vi "Dashboard Main.vi"() -> ()   [LabVIEW 2013]
uses:
  Program Files/National Instruments/LabVIEW 2013/examples/FRC/Vision/2014 Target Detection/TargetType.ctl
  <vilib>/event_ctls.llb/eventvkey.ctl
  <vilib>/Rock Robotics/WPI/Dashboard/WPI_DashboardLogging Global.vi
  <vilib>/Utility/config.llb/Write Key (String).vi
  <vilib>/Utility/config.llb/Write Key (I32).vi
  <vilib>/Utility/config.llb/NI_LVConfig.lvlib
panel:
  out "Image Message":string="Timeout in Camera Communications"
  in  "Rec Mode":enum32{"Stop", "Record", "Playback"}(radio)
  in  "Dashboard Tab":T1(tab)
  in  "Camera Settings":T2={"Frame Rate"=30, "Compression"=30, "Size"=1} {"Frame Rate" scale=1.0..30.0; "Size" items=["640x480", "320x240", "160x120"]}
  out "MotorSliders R":cluster{"MotorSlide1":dbl, "MotorSlide2":dbl} {"MotorSlide2" scale=-1.0..1.0 scale format="%#_2e"; "MotorSlide1" scale=-1.0..1.0 scale format="%#_2e"}
  out "MotorChart R":cluster{"Numeric":dbl, "Numeric":dbl}(graph)
  out "MotorSliders L":T3 {"MotorSlide4 2" scale=0.0..14.0 scale format="%#_2e"; "MotorSlide2" scale=-1.0..1.0 scale format="%#_2e"; "MotorSlide1" scale=-1.0..1.0 scale format="%#_2e"}
  out "MotorChart L":T4(graph)
  out "JS1 Z":dbl(slide) scale=-1.0..1.0 scale format="%#_2e"
  out "Joystick 1":cluster{"X":dbl, "Y":dbl}[](graph)
  out "JS Buttons 1":T5
  out "JS2 Z":dbl(slide) scale=-1.0..1.0 scale format="%#_2e"
  out "Joystick 2":cluster{"X":dbl, "Y":dbl}[](graph)
  out "JS Buttons 2":T5
  out "Mode":T6(ring)=enum."Auto Disabled"
  out "Camera IP":string
  in  "DB Camera Config":bool
  out "fps":dbl format="%#.1g"
  out "Mbps":dbl format="%#.1g"
  out "Mbps 2":bool
  out "LED 1":bool
  in  "Slider 1":dbl(slide) scale=0.0..100.0
  out "Mask":T7(plugin-control)
  out "Distances":T9(array[cluster])
  in  "Score Limit":dbl=70.0
  in  "Color Components":T10={"Hue"={110.0, 142.0}, "Sat"={138.0, 255.0}, "Val"={139.0, 198.0}} {"Val" scale=0.0..255.0; "Sat" scale=0.0..255.0; "Hue" scale=0.0..255.0 scale format="%#_3g"}
  in  "Checkbox 2":bool
  in  "Checkbox 1":bool
  in  "Test Slider":dbl(slide) scale=0.0..100.0 scale format="%#_3g"
  in  "On/Off":bool caption="Solenoid"
  in  "Test Name":u16(ring) items=["Select the test to run...", "Example Test", "-------------------------------", "List of tests is built in robot code.", "Replace with your own automated tests."]
  in  "Test Tree":string(tree)
  in  "Motor":cluster{"Value":dbl, "Enable":bool} {"Value" scale=-1.0..1.0 scale format="%#_3g"}
  out "Progress":T11 {"Test Progress" scale=0.0..100.0}
  in  "Rev/Fwd":cluster{"Forward":bool, "Reverse":bool}
  in  "Test Ring":u16(ring) items=["Auto", "Fixed indoor", "Fixed outdoor 1", "Fixed outdoor 2", "Fixed fluorescent 1", "Fixed fluorescent 2", "Hold current"]
  in  "Listbox":i32(listbox)
  out "Tree":string(tree)
  out "Camera Image":T7(plugin-control)
  in  "Enable":bool
  # "Left"
  # "Front"
  # "Right"
  # "Battery"
  # "Customize by placing controls and indicators here and name to\nmatch Dashboard Variables on robot."
  # "This tab is a great place for autonomous settings and validation.\nCustomize by placing controls and indicators here and name to\nmatch Dashboard Variables on robot."
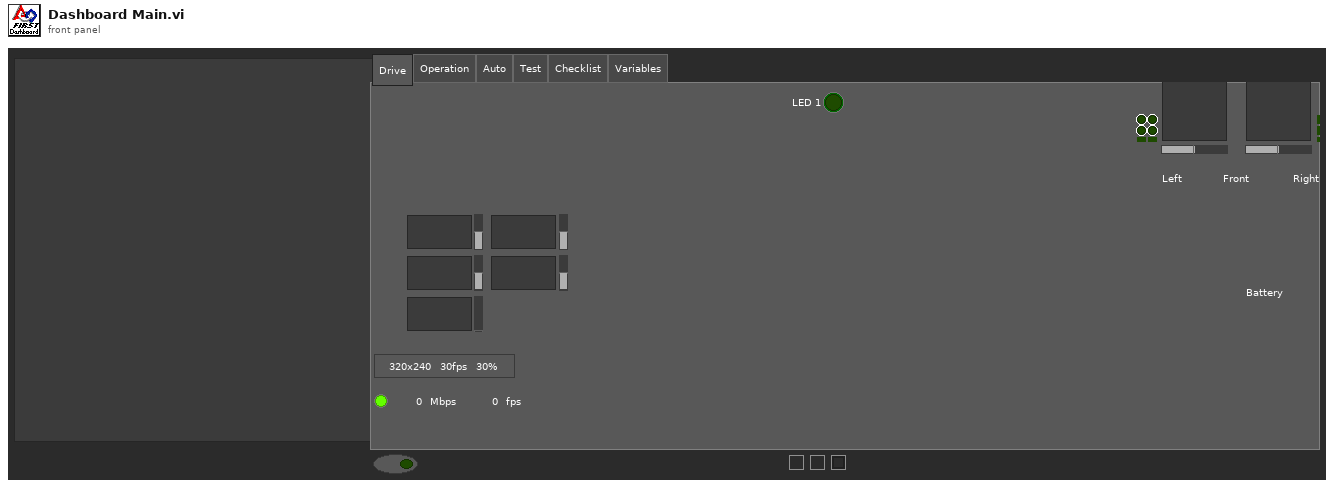
[diagram p1: front panel]
types:
  T1 = enum32{"Drive", "Operation", "Auto", "Test", "Checklist", "Variables"}
  T2 = cluster{"Frame Rate":i32, "Compression":i32, "Size":u16}
  T3 = cluster{"MotorSlide1":dbl, "MotorSlide2":dbl, "MotorSlide4 2":dbl}
  T4 = cluster{"Numeric":dbl, "Numeric":dbl, "Battery":sgl}
  T5 = cluster{bool, bool, bool, bool, bool, bool, bool, bool, bool, bool, bool, bool}
  T6 = enum8{"Tele-Op Disabled", "Tele-Op Enabled", "Auto Disabled", "Auto Enabled", "Test Disabled", "Test Enabled", ""}
  T7 = typedef "IMAQ Image.ctl" = refnum<image>
  T8 = typedef "TargetType.ctl" = enum16{"Not Hot", "Hot"}
  T9 = cluster{"Distance (ft)":dbl, "Target Center (-1 to 1)":cluster{"X":dbl, "Y":dbl}, "Left":bool, "State":T8}[]
  T10 = cluster{"Hue":cluster{dbl, dbl}, "Sat":cluster{dbl, dbl}, "Val":cluster{dbl, dbl}}
  T11 = cluster{"Test Progress":u8, "Test Progress Text":string}
  T12 = typedef "Image Type" = u32
  T13 = cluster{"Horizontal":bool, "Aspect Score":dbl, "Rect Score":dbl, cluster{"Left":dbl, "Top":dbl, "Right":dbl, "Bottom":dbl}, "Equiv H":dbl, "Equiv V":dbl}[]
  T14 = cluster{"Scores":cluster{"Total":dbl, "Left":dbl, "Right":dbl, "Ratio":dbl, "Vertical":dbl, "index":i32, "State":T8}, "Verticals":cluster{"Horizontal?":bool, "Aspect Score":dbl, "Rect Score":dbl, cluster{"Left":dbl, "Top":dbl, "Right":dbl, "Bottom":dbl}, "Equiv H":dbl, "Equiv V":dbl}, "Horizontals":cluster{"Horizontal?":bool, "Aspect Score":dbl, "Rect Score":dbl, cluster{"Left":dbl, "Top":dbl, "Right":dbl, "Bottom":dbl}, "Equiv H":dbl, "Equiv V":dbl}, "Validated":bool}[]
  T15 = cluster{cluster{dbl, dbl}, cluster{dbl, dbl}, cluster{dbl, dbl}}
  T16 = cluster{"Digital Inputs":bool[], "Digital Outputs":bool[]}
  T17 = cluster{"Competition mode":bool, "Robot Link":bool, "Autonomous":bool, "Enabled":bool, "E-Stop":bool, "Simulated":bool, "TestMode":bool, "Docked Window":bool}
  T18 = cluster{"Boolean Array[0]":bool, "Boolean Array[1]":bool, "Boolean Array[2]":bool, "Boolean Array[3]":bool, "Boolean Array[4]":bool, "Boolean Array[5]":bool, "Boolean Array[6]":bool, "Boolean Array[7]":bool, "Boolean Array[8]":bool, "Boolean Array[9]":bool, "Boolean Array[10]":bool, "Boolean Array[11]":bool}
  T19 = typedef "NI_LVConfig.lvlib/Config Data RefNum.ctl" = refnum<k1>
  T20 = typedef "eventvkey.ctl" = enum16{"ASCII", "Enter", "Return", "Shift", "Ctrl", "Alt", "Cmd", "Opt", "Caps", "NumLock", "Clear", "Break", "Up", "Down", "Left", "Right", "Insert", "Delete", "Home", "End", "PageUp", "PageDown", "Escape", "Help", "Pause", "ScrollLock", "F1", "F2", "F3", "F4", "F5", "F6", "F7", "F8", "F9", "F10", "F11", "F12", "F13", "F14", "F15", "F16", "F17", "F18", "F19", "F20", "F21", "F22", "F23", "F24", "Play", "VolumeUp", "VolumeDown", "Mute", "Two Byte Char"}
  T21 = cluster{"Image Size":bool, "Image Type":bool, "Pixel Value":bool, "ROI Information":bool, "Zoom Factor":bool}
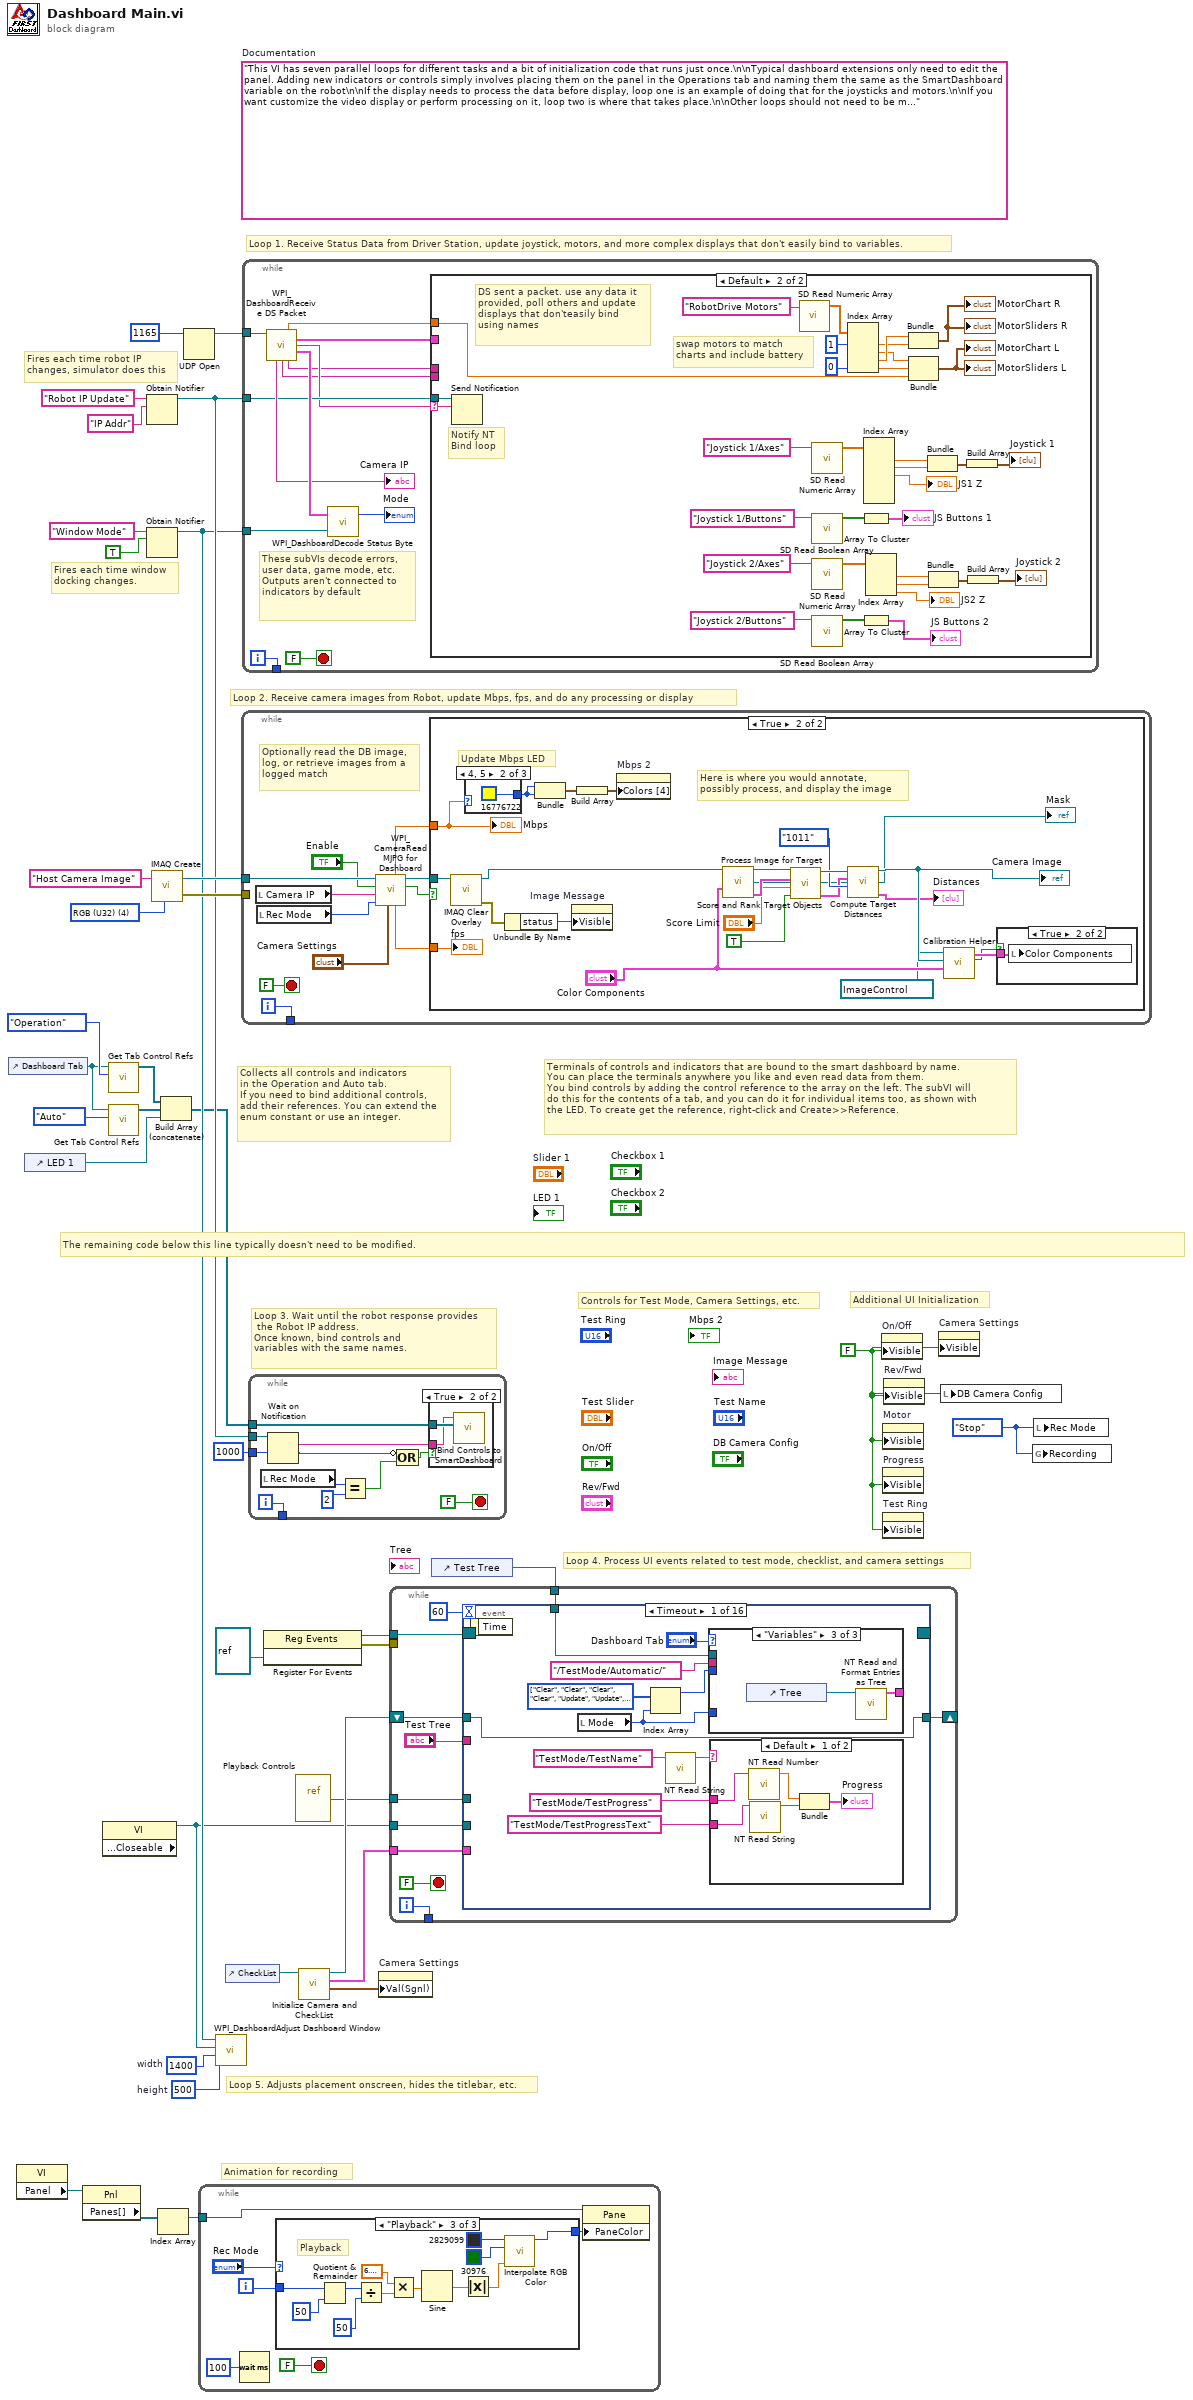
[diagram p0: block diagram]
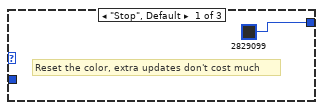
[diagram p2: hidden frame]
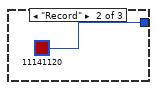
[diagram p3: hidden frame]
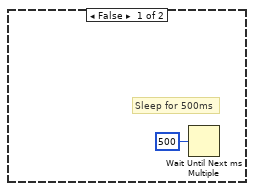
[diagram p5: hidden frame]
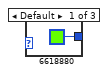
[diagram p7: hidden frame]
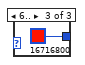
[diagram p8: hidden frame]
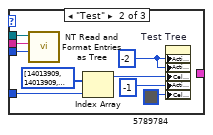
[diagram p10: hidden frame]
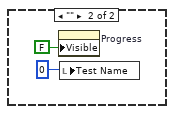
[diagram p11: hidden frame]
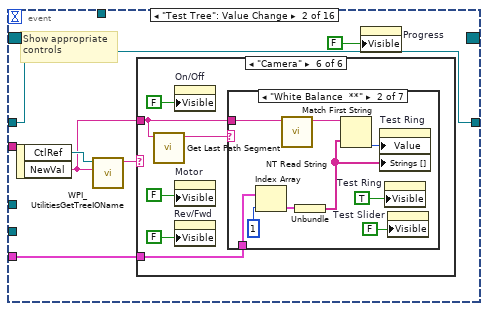
[diagram p12: hidden frame]
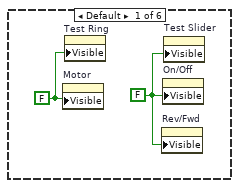
[diagram p13: hidden frame]
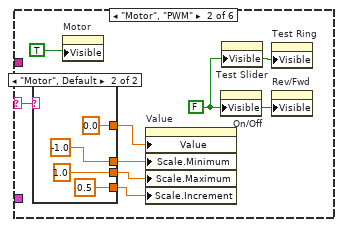
[diagram p14: hidden frame]
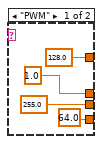
[diagram p15: hidden frame]
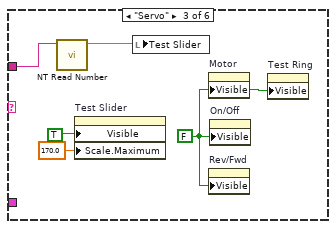
[diagram p16: hidden frame]
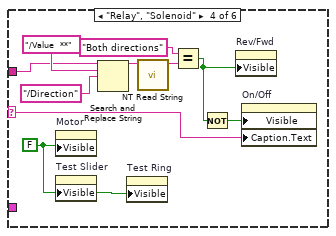
[diagram p17: hidden frame]
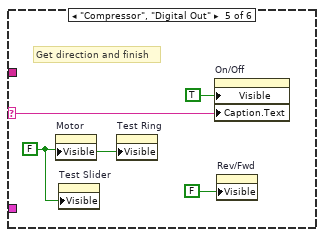
[diagram p18: hidden frame]
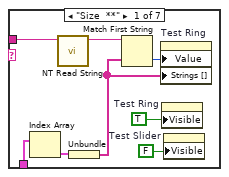
[diagram p19: hidden frame]
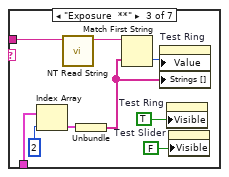
[diagram p20: hidden frame]
diagram:
  w8 = enum32{"Stop", "Record", "Playback"}."Stop" ("Rec Mode")
  w11 = 500  # height
  w12 = 1400  # width
  w25 = FALSE ("Visible")
  (unwired) "This VI has seven parallel loops for different tasks and a bit of initialization code that runs just once.\n\nTypical dashboard extensions only need to edit the panel. Adding new indicators or controls simply involves placing them on the panel in the Operations tab and naming them the same as the SmartDashboard variable on the robot\n\nIf the display needs to process the data before display, loop one is an example of doing that for the joysticks and motors.\n\nIf you want customize the video display or perform processing on it, loop two is where that takes place.\n\nOther loops should not need to be modified. They are pretty standard, and document the task they perform."  # Documentation
  w35 = T12 4 items=["Grayscale (U8)", "Grayscale (I16)", "Grayscale (SGL)", "Complex (CSG)", "RGB (U32)", "HSL (U32)", "RGB (U64)"] ("Image Type")
  # "Controls for Test Mode, Camera Settings, etc."
  # "Additional UI Initialization"
  # "Animation for recording"
  # "Fires each time robot IP\nchanges, simulator does this"
  # "Fires each time window\ndocking changes."
  # "Collects all controls and indicators\nin the Operation and Auto tab.\nIf you need to bind additional controls,\nadd their references. You can extend the\nenum constant or use an integer."
  # "The remaining code below this line typically doesn't need to be modified."
  # "Loop 4. Process UI events related to test mode, checklist, and camera settings"
  # "Terminals of controls and indicators that are bound to the smart dashboard by name.\nYou can place the terminals anywhere you like and even read data from them.\nYou bind controls by adding the control reference to the array on the left. The subVI will\ndo this for the contents of a tab, and you can do it for individual items too, as shown with\nthe LED. To create get the reference, right-click and Create>>Reference."
  # "Loop 3. Wait until the robot response provides\n the Robot IP address.\nOnce known, bind controls and\nvariables with the same names."
  # "Loop 5. Adjusts placement onscreen, hides the titlebar, etc."
  # "Loop 1. Receive Status Data from Driver Station, update joystick, motors, and more complex displays that don't easily bind to variables."
  # "Loop 2. Receive camera images from Robot, update Mbps, fps, and do any processing or display"
  n1 = control-ref of="Dashboard Tab"() -> (w6:refnum<vi>)
  n2 = property class="VI"() -> ("Panel"=w19:refnum<vi>)  [unwired: 2 in, 2 out]
  n3 = control-ref of="LED 1"() -> (w1:refnum<vi>)
  n4 = property class="Pnl"(reference=w19) -> ("Panes[]"=w20:refnum<vi>[])  [unwired: 1 in, 2 out]
  n5 = property class="VI" props=["Front Panel.Closeable"]() -> (reference out=w7:refnum<vi>)  [unwired: 2 in, 2 out]
  n6 = call <vilib>:"Get Tab Control Refs.vi"("Page Index"=T1."Operation" ("Dashboard Tab"), "TabControl in"=w6) -> ("ControlsOnPage"=w4:refnum<vi>[])  [unwired: 9 in]
  n7 = call <vilib>:"Get Tab Control Refs.vi"("Page Index"=T1."Auto" ("Dashboard Tab"), "TabControl in"=w6) -> ("ControlsOnPage"=w5:refnum<vi>[])  [unwired: 9 in]
  n8 = Obtain Notifier(name (unnamed)="Robot IP Update", notification data type="IP Addr" ("name (unnamed)")) -> (notifier out=w29:refnum<notifier>)  [unwired: 2 in, 2 out]
  n9 = Obtain Notifier(name (unnamed)="Window Mode", notification data type=TRUE) -> (notifier out=w10:refnum<notifier>)  [unwired: 2 in, 2 out]
  n10 = call "IMAQ Create"("Image Name"="Host Camera Image", "Image Type"=w35) -> ("New Image"=w33:T7, "error out"=w32:errorcluster)  [unwired: 2 in, 1 out]
  n11 = Index Array(array=w20) -> (element=w18:refnum<vi>)  [unwired: 1 in]
  n12 = Build Array (concatenate)(w4, w5, w1) -> (w3:refnum<vi>[])
  n13 = UDP Open(11:u16 1165 ("port")) -> (port=w36:refnum<k16>)  [unwired: 2 in, 4 out]
  n14 = while {
    tunnel: w18 -> [w39]
    i -> [w42]
    stop <- FALSE stop-if-true
    n15 = Wait (ms)(milliseconds to wait=u32 100) -> ()  [unwired: 1 out]
    n16 = case shown="\"Playback\"" "Rec Mode" {
      tunnel: w42 -> [_ _ w57]
      tunnel: [u32 2829099 ("Base Color") u32 11141120 ("Target Color") w46] -> w38
      frame "Stop", Default {
        # "Reset the color, extra updates don't cost much"
      }
      frame "Record" {
      }
      frame "Playback" {
        # "Playback"
        n17 = Quotient & Remainder(x=w57, y=u32 50 ("milliseconds to wait")) -> (x-y*floor(x/y)=w53:u32)  [unwired: 1 out]
        n18 = Divide(x=w53, y=u32 50 ("milliseconds to wait")) -> (x/y=w50:dbl)
        n19 = Multiply(x=6.283185307179586, y=w50) -> (x*y=w55:dbl)
        n20 = Sine(x=w55) -> (sin(x)=w54:dbl)
        n21 = Absolute Value(x=w54) -> (abs(x)=w47:dbl)
        n22 = call "Interpolate RGB Color.vi"("Proportion"=w47, "Target Color"=u32 30976, "Base Color"=u32 2829099) -> ("Result Color"=w46:u32)  [unwired: 8 in]
      }
    }
    n23 = property class="Pane"(reference=w39, "PaneColor"=w38) -> ()  [unwired: 1 in, 2 out]
  }
  n24 = call <vilib>:"WPI_DashboardAdjust Dashboard Window.vi"("height"=w11, "width"=w12, "reference in"=w7, "Notifier in"=w10) -> ()  [unwired: 8 in]
  n25 = control-ref of="CheckList"() -> (w9:refnum<vi>)
  n26 = while {
    tunnel: w33 -> [w66]
    tunnel: w32 -> [_]
    tunnel: [w67] -> _
    i -> [w67]
    stop <- FALSE stop-if-true
    # "Optionally read the DB image,\nlog, or retrieve images from a\nlogged match"
    n27 = local read "Camera IP"() -> (w59:string)
    n28 = local read "Rec Mode"() -> (w58:enum32{"Stop", "Record", "Playback"})
    n29 = call <vilib>:"WPI_CameraRead MJPG for Dashboard.vi"("Camera Settings"="Camera Settings", "Rec Mode"=w58, "Camera IP"=w59, "Enable"="Enable", "Refnum in"=w66) -> ("Active"=w63:bool, "Refnum out"=w65:T7, "FPS"=w62:dbl, "Bandwidth (Mbps)"=w61:dbl)  [unwired: 3 in]
    n30 = case shown="True" w63 {
      tunnel: w65 -> [_ w87]
      tunnel: w61 -> [_ w86]
      tunnel: w62 -> [_ w85]
      frame False {
        # "Sleep for 500ms"
        n31 = Wait Until Next ms Multiple(millisecond multiple=u32 500) -> ()  [unwired: 1 out]
      }
      frame True {
        # "Here is where you would annotate,\npossibly process, and display the image"
        # "Update Mbps LED"
        n32 = call "IMAQ Clear Overlay"("Image"=w87) -> ("error out"=w91:errorcluster, "Image Out"=w84:T7)  [unwired: 2 in, 7 out]
        n33 = case shown="4, 5" w86 {
          tunnel: [u32 6618880 ("Color Box") u32 16776722 ("Color Box") u32 16716800 ("Color Box")] -> w88
          frame Default {
          }
          frame 4, 5 {
          }
          frame 6.. {
          }
        }
        n34 = Unbundle By Name(w91) -> ("status"=w92:bool)
        n35 = Bundle("Color Box"=w88, "Color Box"=w88) -> (w90:cluster{"Color Box":u32, "Color Box":u32})  [unwired: 1 out]
        n36 = property on="Image Message" class="Str"("Visible"=w92) -> ()  [unwired: 2 in, 2 out]
        n37 = Build Array(w90) -> (w89:cluster{"Color Box":u32, "Color Box":u32}[])
        n38 = property on="Mbps 2" class="Bool (strict)"("Colors [4]"=w89) -> ()  [unwired: 2 in, 2 out]
        n39 = call "Process Image for Target.vi"("Src Image"=w84, "Color Components"="Color Components") -> ("Src Image Out"=w83:T7, "Threshold"=→"Mask":T7, "Particles"=w78:T13)  [unwired: 11 in]
        n40 = call "Score and Rank Target Objects.vi"("Annotate"=TRUE, "Score Limit"="Score Limit", "Particles"=w78, "Image in"=w83) -> ("Target Info"=w73:T14, "Annotated Image"=w82:T7)  [unwired: 6 in]
        n41 = call "Compute Target Distances.vi"("Camera Type"=enum16{"206", "1011", "1013"}."1011", "Target Info"=w73, "Image in"=w82) -> ("Distances"=→"Distances":T9, "Image out"=w81:T7)  [unwired: 6 in, 1 out]
        "Camera Image" <- w81
        n42 = call "Calibration Helper.vi"("Color Components"="Color Components", "Image"=w81, "Image Ctl Refnum"=refnum<vi> refnum) -> ("Changed"=w71:bool, "output color"=w79:T15)  [unwired: 7 in]
        n43 = case shown="True" w71 {
          tunnel: w79 -> [_ w93]
          frame False {
          }
          frame True {
            n44 = local write "Color Components"(w93) -> ()
          }
        }
        "Mbps" <- w86
        "fps" <- w85
      }
    }
  }
  n45 = while {
    tunnel: w36 -> [w107]
    tunnel: w29 -> [w102]
    tunnel: w10 -> [w106]
    tunnel: [w103] -> _
    i -> [w103]
    stop <- FALSE stop-if-true
    # "These subVIs decode errors, user data, game mode, etc.\nOutputs aren't connected to indicators by default"
    n46 = call <vilib>:"WPI_DashboardReceive DS Packet.vi"("Recv Socket"=w107) -> ("Battery"=w97:sgl, "Driver Station"=w98:T16, "Robot IP Address"=w101:string, "Status"=w108:T17, "Camera IP Address"=→"Camera IP":string, "Low Priority User Data"=w100:string, "High Priority User Data"=w99:string)  [unwired: 1 in, 7 out]
    n47 = call <vilib>:"WPI_DashboardDecode Status Byte.vi"("Window Mode Notifier"=w106, "Status"=w108) -> ("Mode"=→"Mode":T6)  [unwired: 1 out]
    n48 = case shown="Default" w101 {
      selector: w101 -> [_ w120]
      tunnel: w102 -> [_ w121]
      tunnel: w100 -> [_ _]
      tunnel: w99 -> [_ _]
      tunnel: w98 -> [_ _]
      tunnel: w97 -> [_ w119]
      frame "0.0.0.0" {
        # "DS not sending packets, or no robot exists yet.\nDon't poll the variables"
      }
      frame Default {
        # "Notify NT\nBind loop"
        # "DS sent a packet. use any data it\nprovided, poll others and update\ndisplays that don'teasily bind\nusing names"
        # "swap motors to match\ncharts and include battery"
        n49 = Send Notification(notification=w120, notifier=w121) -> ()  [unwired: 1 in, 2 out]
        n50 = call <vilib>:"SD Read Numeric Array.vi"("Name"="RobotDrive Motors") -> ("Numeric Array"=w118:dbl[])  [unwired: 8 in, 2 out]
        n51 = call <vilib>:"SD Read Numeric Array.vi"("Name"="Joystick 1/Axes") -> ("Numeric Array"=w137:dbl[])  [unwired: 8 in, 2 out]
        n52 = call <vilib>:"SD Read Boolean Array.vi"("Name"="Joystick 1/Buttons") -> ("Boolean Array"=w139:bool[])  [unwired: 8 in, 2 out]
        n53 = call <vilib>:"SD Read Numeric Array.vi"("Name"="Joystick 2/Axes") -> ("Numeric Array"=w131:dbl[])  [unwired: 8 in, 2 out]
        n54 = call <vilib>:"SD Read Boolean Array.vi"("Name"="Joystick 2/Buttons") -> ("Boolean Array"=w130:bool[])  [unwired: 8 in, 2 out]
        n55 = Index Array(array=w118, index #1=1, index #4=0) -> (element #1=w114:dbl, element #2=w113:dbl, element #3=w115:dbl, element #4=w110:dbl)  [unwired: 2 in]
        n56 = Array To Cluster(array=w139) -> (cluster=→"JS Buttons 1":T18)
        n57 = Array To Cluster(array=w130) -> (cluster=→"JS Buttons 2":T18)
        n58 = Index Array(array=w137) -> (element #1=w134:dbl, element #2=w135:dbl, element #3=→"JS1 Z":dbl)  [unwired: 6 in, 3 out]
        n59 = Index Array(array=w131) -> (element #1=w126:dbl, element #2=w125:dbl, element #3=→"JS2 Z":dbl)  [unwired: 3 in]
        n60 = Bundle("Numeric"=w115, "Numeric"=w114) -> (→"MotorChart R" →"MotorSliders R":cluster{"Numeric":dbl, "Numeric":dbl})  [unwired: 1 in]
        n61 = Bundle("Numeric"=w113, "Numeric"=w110, "Battery"=w119) -> (→"MotorChart L" →"MotorSliders L":T4)  [unwired: 1 in]
        n62 = Bundle("Numeric"=w134, "Numeric"=w135) -> (w133:cluster{"Numeric":dbl, "Numeric":dbl})  [unwired: 1 in]
        n63 = Bundle("Numeric"=w126, "Numeric"=w125) -> (w127:cluster{"Numeric":dbl, "Numeric":dbl})  [unwired: 1 in]
        n64 = Build Array(w133) -> (→"Joystick 1":cluster{"Numeric":dbl, "Numeric":dbl}[])
        n65 = Build Array(w127) -> (→"Joystick 2":cluster{"Numeric":dbl, "Numeric":dbl}[])
      }
    }
  }
  n66 = while {
    tunnel: w3 -> [w153]
    tunnel: w29 -> [w151]
    tunnel: [w149] -> _
    tunnel: u32 1000 ("milliseconds to wait") -> [w148]
    i -> [w149]
    stop <- FALSE stop-if-true
    n67 = local read "Rec Mode"() -> (w144:enum32{"Stop", "Record", "Playback"})
    n68 = Wait on Notification(notifier=w151, timeout in ms (-1)=w148) -> (notification=w150:string, timed out?=w146:bool)  [unwired: 2 in, 2 out]
    n69 = Equal?(x=w144, y=u16 2 ("Rec Mode")) -> (x = y?=w145:bool)
    n70 = Compound Arithmetic op=OR(invert w146, w145) -> (w147:bool)
    n71 = case shown="True" w147 {
      tunnel: w153 -> [_ w155]
      tunnel: w150 -> [_ w154]
      frame False {
      }
      frame True {
        n72 = call <vilib>:"Bind Controls to SmartDashboard.vi"("Bound Control Refs"=w155, "Server IP Address"=w154) -> ()  [unwired: 10 in]
      }
    }
  }
  n73 = register-events(refnum<vi> refnum) -> (reference out=w16:refnum<event-registration>, error out=w15:errorcluster)  [unwired: 2 in]
  n74 = vi-ref "Playback Controls.vi"() -> (w17:refnum<vi>)
  n75 = call "Initialize Camera and CheckList.vi"("ListBox in"=w9) -> ("Cluster"=w23:cluster{"value":i32, "value":i32, "index":i32}, "Array"=w24:cluster{string[]}[], "File Refnum"=w22:T19)  [unwired: 8 in]
  n76 = property on="Camera Settings" class="Clust (strict)"("Val(Sgnl)"=w23) -> ()  [unwired: 2 in, 2 out]
  n77 = control-ref of="Test Tree"() -> (w21:refnum<vi>)
  n78 = while {
    tunnel: w24 -> [w163]
    shift-right: [w162] -> _
    shift-left: w22 -> [w161]
    tunnel: [w160] -> _
    tunnel: w21 -> [w159]
    tunnel: w17 -> [w158]
    tunnel: w16 -> [w157]
    tunnel: w15 -> [_]
    tunnel: w7 -> [w156]
    i -> [w160]
    stop <- FALSE stop-if-true
    n79 = event shown="[0] Timeout" {
      selector: w157 -> [_ _ _ _ _ _ _ _ _ _ _ _ _ _ _ _]
      dyn-events: [_ _ _ _ _ _ _ _ _ _ _ _ _ w401 _ _] -> _
      timeout: u32 60 ("milliseconds to wait") -> [_ _ _ _ _ _ _ _ _ _ _ _ _ _ _ _]
      tunnel: w159 -> [w173 _ _ _ _ _ _ _ _ _ _ _ _ _ _ _]
      tunnel: "Test Tree" -> [_ _ _ _ _ _ _ _ w370 w378 w380 w384 w392 _ _ _]
      tunnel: w163 -> [_ w197 _ _ _ _ w334 w364 _ _ _ _ _ _ _ _]
      tunnel: [w167 w196 w295 w300 w308 w320 w333 w357 w369 w376 w379 w383 w391 w403 w417 w418] -> w162
      tunnel: w161 -> [w167 w196 w295 w300 w308 w320 w332 w357 w369 w376 w379 w383 w391 w403 w417 w418]
      tunnel: w158 -> [_ _ _ _ _ _ _ _ _ _ _ _ _ w404 _ w421]
      tunnel: w156 -> [_ _ _ _ _ _ _ _ _ _ _ _ _ w399 _ _]
      event Timeout {
        w172 = enum16{"Update", "Clear"}[] [enum."Clear", enum."Clear", enum."Clear", enum."Clear", enum."Update", enum."Update", enum."Clear"] items=["Update", "Clear"]
        n80 = event-data() -> ()  [unwired: 1 in, 1 out]
        n81 = local read "Mode"() -> (w170:T6)
        n82 = Index Array(array=w172, index=w170) -> (element=w171:enum16{"Update", "Clear"})
        n83 = call <vilib>:"NT Read String.vi"("Name"="TestMode/TestName") -> ("String"=w176:string)  [unwired: 9 in, 1 out]
        n84 = case shown="\"Variables\"" "Dashboard Tab" {
          tunnel: w173 -> [_ w186 _]
          tunnel: "/TestMode/Automatic/" ("Name Pattern") -> [_ w185 _]
          tunnel: w171 -> [_ w184 _]
          tunnel: w170 -> [_ w182 _]
          tunnel: [_ _ w188] -> _
          frame "Operation", Default {
          }
          frame "Test" {
            w181 = -2 ("Active Item:Row Number")
            n85 = call <vilib>:"NT Read and Format Entries as Tree.vi"("Operation"=w184, "Name Pattern"=w185, "Tree Refnum"=w186) -> ()  [unwired: 7 in, 2 out]
            n86 = Index Array(array=u32[] [14013909, 14013909, 14013909, 14013909, 14013909, 16777215, 14013909], index=w182) -> (element=w180:u32)
            n87 = property on="Test Tree" class="Tree (strict)"("Active Item Row Number"=w181, "ActiveColNum"=w181, "CellBG"=w180, "Active Item Row Number"=-1 ("Active Item:Row Number"), "CellBG"=u32 5789784 ("Color Box")) -> ()  [unwired: 2 in, 2 out]
          }
          frame "Variables" {
            n88 = control-ref of="Tree"() -> (w187:refnum<vi>)
            n89 = call <vilib>:"NT Read and Format Entries as Tree.vi"("Tree Refnum"=w187) -> ("Formatted Strings"=w188:cluster{"Name":string, "Value":string}[])  [unwired: 9 in, 1 out]
          }
        }
        n90 = case shown="Default" w176 {
          tunnel: "TestMode/TestProgress" ("Name") -> [w190 _]
          tunnel: "TestMode/TestProgressText" ("Name") -> [w189 _]
          frame Default {
            n91 = call <vilib>:"NT Read Number.vi"("Name"=w190) -> ("Numeric"=w191:dbl)  [unwired: 9 in, 1 out]
            n92 = call <vilib>:"NT Read String.vi"("Name"=w189) -> ("String"=w192:string)  [unwired: 9 in, 1 out]
            n93 = Bundle("Numeric"=w191, "String"=w192) -> (→"Progress":cluster{"Numeric":dbl, "String":string})  [unwired: 1 in]
          }
          frame "" {
            n94 = property on="Progress" class="Clust (strict)"("Visible"=FALSE) -> ()  [unwired: 2 in, 2 out]
            n95 = local write "Test Name"(u16 0) -> ()
          }
        }
      }
      event "Test Tree": Value Change {
        # "Show appropriate\ncontrols"
        n96 = event-data() -> ("CtlRef"=w200:refnum<vi>, "NewVal"=w198:string)  [unwired: 1 in]
        n97 = call <vilib>:"WPI_UtilitiesGetTreeIOName.vi"("NewVal"=w198, "TreeControl in"=w200) -> ("I/O Name"=w201:string)  [unwired: 9 in]
        n98 = case shown="\"Camera\"" w201 {
          selector: w201 -> [_ w208 _ w226 w235 _]
          tunnel: w198 -> [_ _ w223 w225 _ w242]
          tunnel: w197 -> [_ _ _ _ _ w241]
          frame Default {
            w203 = FALSE ("Visible")
            w202 = FALSE ("Visible")
            n99 = property on="Motor" class="Clust (strict)"("Visible"=w202) -> ()  [unwired: 2 in, 2 out]
            n100 = property on="Test Ring" class="Ring (strict)"("Visible"=w202) -> ()  [unwired: 2 in, 2 out]
            n101 = property on="Rev/Fwd" class="Clust (strict)"("Visible"=w203) -> ()  [unwired: 2 in, 2 out]
            n102 = property on="On/Off" class="Bool (strict)"("Visible"=w203) -> ()  [unwired: 2 in, 2 out]
            n103 = property on="Test Slider" class="Slide (strict)"("Visible"=w203) -> ()  [unwired: 2 in, 2 out]
          }
          frame "Motor", "PWM" {
            w209 = FALSE ("Visible")
            n104 = case shown="\"Motor\", Default" w208 {
              tunnel: [1.0 ("Value") -1.0 ("Value")] -> w207
              tunnel: [255.0 ("Value") 1.0 ("Value")] -> w206
              tunnel: [128.0 ("Value") 0.0 ("Value")] -> w205
              tunnel: [64.0 ("Value") 0.5 ("Value")] -> w204
              frame "PWM" {
              }
              frame "Motor", Default {
              }
            }
            n105 = property on="Motor" class="Clust (strict)"("Visible"=TRUE) -> ()  [unwired: 2 in, 2 out]
            n106 = property on="Value" class="Slide (strict)"("Value"=w205, "Scale.Minimum"=w207, "Scale.Maximum"=w206, "Scale.Increment"=w204) -> ()  [unwired: 2 in, 2 out]
            n107 = property on="On/Off" class="Bool (strict)"("Visible"=w209) -> ()  [unwired: 2 in, 2 out]
            n108 = property on="Test Slider" class="Slide (strict)"("Visible"=w209) -> ()  [unwired: 2 in, 2 out]
            n109 = property on="Test Ring" class="Ring (strict)"("Visible"=w209) -> ()  [unwired: 2 in, 2 out]
            n110 = property on="Rev/Fwd" class="Clust (strict)"("Visible"=w209) -> ()  [unwired: 2 in, 2 out]
          }
          frame "Servo" {
            w221 = FALSE ("Visible")
            n111 = call <vilib>:"NT Read Number.vi"("Name"=w223) -> ("Numeric"=w222:dbl)  [unwired: 9 in, 1 out]
            n112 = property on="Test Slider" class="Slide (strict)"("Visible"=TRUE, "Scale.Maximum"=170.0 ("Scale.Range:Maximum")) -> ()  [unwired: 2 in, 2 out]
            n113 = local write "Test Slider"(w222) -> ()
            n114 = property on="Motor" class="Clust (strict)"("Visible"=w221) -> ()  [unwired: 2 in, 2 out]
            n115 = property on="Rev/Fwd" class="Clust (strict)"("Visible"=w221) -> ()  [unwired: 2 in, 2 out]
            n116 = property on="On/Off" class="Bool (strict)"("Visible"=w221) -> ()  [unwired: 2 in, 2 out]
            n117 = property on="Test Ring" class="Ring (strict)"("Visible"=w221) -> ()  [unwired: 2 in, 2 out]
          }
          frame "Relay", "Solenoid" {
            w224 = FALSE ("Visible")
            n118 = property on="Motor" class="Clust (strict)"("Visible"=w224) -> ()  [unwired: 2 in, 2 out]
            n119 = property on="Test Slider" class="Slide (strict)"("Visible"=w224) -> ()  [unwired: 2 in, 2 out]
            n120 = Search and Replace String(input string=w225, search string="/Value  **", replace string="/Direction") -> (result string=w231:string)  [unwired: 5 in, 3 out]
            n121 = property on="Test Ring" class="Ring (strict)"("Visible"=w224) -> ()  [unwired: 2 in, 2 out]
            n122 = call <vilib>:"NT Read String.vi"("Name"=w231) -> ("String"=w229:string)  [unwired: 9 in, 1 out]
            n123 = Equal?(x="Both directions", y=w229) -> (x = y?=w227:bool)
            n124 = Not(x=w227) -> (.not. x?=w228:bool)
            n125 = property on="Rev/Fwd" class="Clust (strict)"("Visible"=w227) -> ()  [unwired: 2 in, 2 out]
            n126 = property on="On/Off" class="Bool (strict)"("Visible"=w228, "Caption.Text"=w226) -> ()  [unwired: 2 in, 2 out]
          }
          frame "Compressor", "Digital Out" {
            w234 = FALSE ("Visible")
            # "Get direction and finish"
            n127 = property on="Motor" class="Clust (strict)"("Visible"=w234) -> ()  [unwired: 2 in, 2 out]
            n128 = property on="Test Slider" class="Slide (strict)"("Visible"=w234) -> ()  [unwired: 2 in, 2 out]
            n129 = property on="Test Ring" class="Ring (strict)"("Visible"=w234) -> ()  [unwired: 2 in, 2 out]
            n130 = property on="On/Off" class="Bool (strict)"("Visible"=TRUE, "Caption.Text"=w235) -> ()  [unwired: 2 in, 2 out]
            n131 = property on="Rev/Fwd" class="Clust (strict)"("Visible"=FALSE) -> ()  [unwired: 2 in, 2 out]
          }
          frame "Camera" {
            n132 = call <vilib>:"Get Last Path Segment.vi"("String in"=w242) -> ("String out"=w243:string)  [unwired: 10 in]
            n133 = property on="On/Off" class="Bool (strict)"("Visible"=FALSE) -> ()  [unwired: 2 in, 2 out]
            n134 = property on="Motor" class="Clust (strict)"("Visible"=FALSE) -> ()  [unwired: 2 in, 2 out]
            n135 = property on="Rev/Fwd" class="Clust (strict)"("Visible"=FALSE) -> ()  [unwired: 2 in, 2 out]
            n136 = case shown="\"White Balance  **\"" w243 {
              tunnel: w242 -> [w249 w258 w267 w276 w285 _ w291]
              tunnel: w241 -> [w247 w255 w264 w273 w282 _ _]
              frame "Size  **" {
                n137 = Index Array(array=w247) -> (element=w246:cluster{string[]})  [unwired: 1 in]
                n138 = call <vilib>:"NT Read String.vi"("Name"=w249) -> ("String"=w248:string)  [unwired: 9 in, 1 out]
                n139 = Unbundle(w246) -> (w244:string[])
                n140 = Match First String(2:w244, 3:w248) -> (0:w245:i32)  [unwired: 1 out]
                n141 = property on="Test Ring" class="Ring (strict)"("Value"=w245, "Strings []"=w244) -> ()  [unwired: 2 in, 2 out]
                n142 = property on="Test Ring" class="Ring (strict)"("Visible"=TRUE) -> ()  [unwired: 2 in, 2 out]
                n143 = property on="Test Slider" class="Slide (strict)"("Visible"=FALSE) -> ()  [unwired: 2 in, 2 out]
              }
              frame "White Balance  **" {
                n144 = Index Array(array=w255, index=1) -> (element=w256:cluster{string[]})
                n145 = call <vilib>:"NT Read String.vi"("Name"=w258) -> ("String"=w257:string)  [unwired: 9 in, 1 out]
                n146 = Unbundle(w256) -> (w253:string[])
                n147 = Match First String(2:w253, 3:w257) -> (0:w252:i32)  [unwired: 1 out]
                n148 = property on="Test Ring" class="Ring (strict)"("Value"=w252, "Strings []"=w253) -> ()  [unwired: 2 in, 2 out]
                n149 = property on="Test Ring" class="Ring (strict)"("Visible"=TRUE) -> ()  [unwired: 2 in, 2 out]
                n150 = property on="Test Slider" class="Slide (strict)"("Visible"=FALSE) -> ()  [unwired: 2 in, 2 out]
              }
              frame "Exposure  **" {
                n151 = Index Array(array=w264, index=2) -> (element=w265:cluster{string[]})
                n152 = call <vilib>:"NT Read String.vi"("Name"=w267) -> ("String"=w266:string)  [unwired: 9 in, 1 out]
                n153 = Unbundle(w265) -> (w261:string[])
                n154 = Match First String(2:w261, 3:w266) -> (0:w262:i32)  [unwired: 1 out]
                n155 = property on="Test Ring" class="Ring (strict)"("Value"=w262, "Strings []"=w261) -> ()  [unwired: 2 in, 2 out]
                n156 = property on="Test Ring" class="Ring (strict)"("Visible"=TRUE) -> ()  [unwired: 2 in, 2 out]
                n157 = property on="Test Slider" class="Slide (strict)"("Visible"=FALSE) -> ()  [unwired: 2 in, 2 out]
              }
              frame "Exposure Priority  **" {
                n158 = Index Array(array=w273, index=3) -> (element=w274:cluster{string[]})
                n159 = call <vilib>:"NT Read String.vi"("Name"=w276) -> ("String"=w275:string)  [unwired: 9 in, 1 out]
                n160 = Unbundle(w274) -> (w270:string[])
                n161 = Match First String(2:w270, 3:w275) -> (0:w271:i32)  [unwired: 1 out]
                n162 = property on="Test Ring" class="Ring (strict)"("Value"=w271, "Strings []"=w270) -> ()  [unwired: 2 in, 2 out]
                n163 = property on="Test Ring" class="Ring (strict)"("Visible"=TRUE) -> ()  [unwired: 2 in, 2 out]
                n164 = property on="Test Slider" class="Slide (strict)"("Visible"=FALSE) -> ()  [unwired: 2 in, 2 out]
              }
              frame "Color Enable  **" {
                n165 = Index Array(array=w282, index=4) -> (element=w283:cluster{string[]})
                n166 = call <vilib>:"NT Read String.vi"("Name"=w285) -> ("String"=w284:string)  [unwired: 9 in, 1 out]
                n167 = Unbundle(w283) -> (w279:string[])
                n168 = Match First String(2:w279, 3:w284) -> (0:w280:i32)  [unwired: 1 out]
                n169 = property on="Test Ring" class="Ring (strict)"("Value"=w280, "Strings []"=w279) -> ()  [unwired: 2 in, 2 out]
                n170 = property on="Test Ring" class="Ring (strict)"("Visible"=TRUE) -> ()  [unwired: 2 in, 2 out]
                n171 = property on="Test Slider" class="Slide (strict)"("Visible"=FALSE) -> ()  [unwired: 2 in, 2 out]
              }
              frame Default {
                n172 = property on="Test Ring" class="Ring (strict)"("Visible"=FALSE) -> ()  [unwired: 2 in, 2 out]
                n173 = property on="Test Slider" class="Slide (strict)"("Visible"=FALSE) -> ()  [unwired: 2 in, 2 out]
              }
              frame "Brightness  **", "Color Level  **", "Compression  **", "FPS  **", "Sharpness  **" {
                n174 = call <vilib>:"NT Read Number.vi"("Name"=w291) -> ("Numeric"=w290:dbl)  [unwired: 9 in, 1 out]
                n175 = local write "Test Slider"(w290) -> ()
                n176 = property on="Test Slider" class="Slide (strict)"("Visible"=TRUE, "Scale.Maximum"=100.0 ("Scale.Range:Maximum")) -> ()  [unwired: 2 in, 2 out]
                n177 = property on="Test Ring" class="Ring (strict)"("Visible"=FALSE) -> ()  [unwired: 2 in, 2 out]
              }
            }
          }
        }
        n178 = property on="Progress" class="Clust (strict)"("Visible"=FALSE) -> ()  [unwired: 2 in, 2 out]
      }
      event "Test Name": Mouse Enter {
        # "Populate the ring with the list of tests"
        n179 = event-data() -> ()  [unwired: 1 in, 1 out]
        n180 = call <vilib>:"NT Read String Array.vi"("Name"="TestMode/TestList") -> ("String Array"=w299:string[])  [unwired: 9 in, 1 out]
        n181 = Build Array (concatenate)("Select the test to run...", w299) -> (w298:string[])
        n182 = property on="Test Name" class="Ring (strict)"("Strings []"=w298) -> ()  [unwired: 2 in, 2 out]
      }
      event "Test Name": Value Change {
        w301 = FALSE ("Visible")
        # "Tell the robot the test name to run"
        n183 = event-data() -> ("NewVal"=w305:u16)  [unwired: 1 in]
        n184 = property on="Test Name" class="Ring (strict)"() -> ("Strings []"=w306:string[])  [unwired: 2 in, 2 out]
        n185 = local write "Progress"(T11 {"Test Progress"=0, "Test Progress Text"=""} ("Progress")) -> ()
        n186 = Index Array(array=w306, index=w305) -> (element=w304:string)
        n187 = call <vilib>:"NT Write String.vi"("String"=w304, "Name"="TestMode/TestName") -> ()  [unwired: 9 in, 1 out]
        n188 = property on="Progress" class="Clust (strict)"("Visible"=TRUE) -> ()  [unwired: 2 in, 2 out]
        n189 = property on="Motor" class="Clust (strict)"("Visible"=w301) -> ()  [unwired: 2 in, 2 out]
        n190 = property on="Test Slider" class="Slide (strict)"("Visible"=w301) -> ()  [unwired: 2 in, 2 out]
        n191 = property on="On/Off" class="Bool (strict)"("Visible"=w301) -> ()  [unwired: 2 in, 2 out]
        n192 = property on="Rev/Fwd" class="Clust (strict)"("Visible"=w301) -> ()  [unwired: 2 in, 2 out]
        n193 = property on="Test Ring" class="Ring (strict)"("Visible"=w301) -> ()  [unwired: 2 in, 2 out]
      }
      event "Listbox": Double Click {
        n194 = event-data() -> ("PlatMods.Shift"=w309:bool, "Row"=w311:i32)  [unwired: 1 in]
        n195 = case shown="True" w309 {
          tunnel: w311 -> [w315 _]
          tunnel: 1 -> [w314 _]
          frame False {
            n196 = property on="Listbox" class="LstBox (strict)"() -> ("Item Symbols"=w313:i32[])  [unwired: 2 in, 2 out]
            n197 = Replace Array Subset(array=w313, new element=w314, index=w315) -> (w312:i32[])
            n198 = property on="Listbox" class="LstBox (strict)"("Item Symbols"=w312) -> ()  [unwired: 2 in, 2 out]
          }
          frame True {
            w316 = 0 ("Top Row")
            n199 = property on="Listbox" class="LstBox (strict)"() -> ("Number of Rows"=w318:u32)  [unwired: 2 in, 2 out]
            n200 = Initialize Array(0, w318) -> (w317:i32[])
            n201 = property on="Listbox" class="LstBox (strict)"("Top Row"=w316, "Value"=w316, "Item Symbols"=w317) -> ()  [unwired: 2 in, 2 out]
          }
        }
      }
      event "Listbox": Key Down {
        n202 = event-data() -> ("VKey"=w322:T20)  [unwired: 1 in]
        n203 = case shown="\"Left\", \"Right\"" w322 {
          selector: w322 -> [w327 _]
          tunnel: eventvkey."Left" ("VKey") -> [w325 _]
          frame "Left", "Right" {
            n204 = Equal?(x=w325, y=w327) -> (x = y?=w326:bool)
            n205 = Select(t=0, s=w326, f=1) -> (s? t:f=w328:i32)
            n206 = property on="Listbox" class="LstBox (strict)"() -> ("Item Symbols"=w331:i32[])  [unwired: 2 in, 2 out]
            n207 = Replace Array Subset(array=w331, new element=w328, index="Listbox") -> (w330:i32[])
            n208 = property on="Listbox" class="LstBox (strict)"("Item Symbols"=w330) -> ()  [unwired: 2 in, 2 out]
          }
          frame Default {
          }
        }
      }
      event "DB Camera Config": Value Change {
        n209 = event-data() -> ("NewVal"=w335:bool)  [unwired: 1 in]
        n210 = case shown="False" w335 {
          tunnel: w334 -> [w344 _]
          tunnel: [w337 w355] -> w333
          tunnel: w332 -> [w336 w355]
          frame False {
            w351 = "Camera"
            w354 = FALSE ("Visible")
            n211 = local read "Camera Settings"() -> (w343:T2)
            n212 = Index Array(array=w344) -> (element=w347:cluster{string[]})  [unwired: 1 in]
            n213 = Unbundle(w343) -> ("Frame Rate"=w342:i32, "Compression"=w341:i32, "Size"=w345:u16)
            n214 = Unbundle(w347) -> (w346:string[])
            n215 = Index Array(array=w346, index=w345) -> (element=w340:string)
            n216 = call-poly <vilib>:"Write Key.vi"("section"=w351, "value"=w340, "key"="Size", "refnum"=w336) -> ("refnum out"=w353:T19)  [unwired: 2 in, 5 out]
            n217 = call-poly <vilib>:"Write Key.vi"("section"=w351, "value"=w342, "key"="FrameRate", "refnum"=w353) -> ("refnum out"=w352:T19)  [unwired: 1 in, 6 out]
            n218 = property on="Camera Settings" class="Clust (strict)"("Visible"=w354) -> ()  [unwired: 2 in, 2 out]
            n219 = local write "DB Camera Config"(w354) -> ()
            n220 = call-poly <vilib>:"Write Key.vi"("section"=w351, "value"=w341, "key"="Compression", "refnum"=w352) -> ("refnum out"=w338:T19)  [unwired: 1 in, 6 out]
            n221 = call <vilib>:"Close Config Data.vi"("refnum"=w338) -> ("file path"=w339:path)  [unwired: 2 in, 8 out]
            n222 = call <vilib>:"Open Config Data.vi"("configuration file path"=w339) -> ("refnum"=w337:T19)  [unwired: 8 in, 2 out]
          }
          frame True {
            n223 = property on="Camera Settings" class="Clust (strict)"("Visible"=TRUE) -> ()  [unwired: 2 in, 2 out]
          }
        }
      }
      event "Camera Settings": Value Change {
        n224 = event-data() -> ("NewVal"=w368:T2)  [unwired: 1 in]
        n225 = Index Array(array=w364) -> (element=w363:cluster{string[]})  [unwired: 1 in]
        n226 = Unbundle(w368) -> ("Frame Rate"=w359:i32, "Compression"=w358:i32, "Size"=w361:u16)
        n227 = Unbundle(w363) -> (w362:string[])
        n228 = Index Array(array=w362, index=w361) -> (element=w360:string)
        n229 = Format Into String(format string="%s   %dfps   %d%%", w360, w359, w358) -> (resulting string=w365:string)  [unwired: 2 in, 1 out]
        n230 = Build Array(w365) -> (w366:string[])
        n231 = property on="DB Camera Config" class="Bool (strict)"("Strings [4]"=w366) -> ()  [unwired: 2 in, 2 out]
      }
      event "Motor.Enable": Value Change {
        n232 = event-data() -> ("NewVal"=w374:bool)  [unwired: 1 in]
        n233 = Unbundle("Motor") -> ("Value"=w373:dbl)  [unwired: 1 out]
        n234 = Select(t=w373, s=w374, f=0.0) -> (s? t:f=w371:dbl)
        n235 = call <vilib>:"NT Write Number.vi"("Numeric"=w371, "Name"=w370) -> ()  [unwired: 9 in, 1 out]
      }
      event "Test Slider": Value Change {
        n236 = event-data() -> ("NewVal"=w377:dbl)  [unwired: 1 in]
        n237 = call <vilib>:"NT Write Number.vi"("Numeric"=w377, "Name"=w378) -> ()  [unwired: 9 in, 1 out]
      }
      event "On/Off": Value Change {
        n238 = event-data() -> ("NewVal"=w382:bool)  [unwired: 1 in]
        n239 = Boolean To (0,1)(Boolean=w382) -> (0, 1=w381:i16)
        n240 = call <vilib>:"NT Write Number.vi"("Numeric"=w381, "Name"=w380) -> ()  [unwired: 9 in, 1 out]
      }
      event "Rev/Fwd": Value Change {
        n241 = event-data() -> ("NewVal.Forward"=w390:bool, "NewVal.Reverse"=w389:bool)  [unwired: 1 in]
        n242 = Boolean To (0,1)(Boolean=w390) -> (0, 1=w386:i16)
        n243 = Boolean To (0,1)(Boolean=w389) -> (0, 1=w388:i16)
        n244 = Negate(x=w388) -> (-x=w387:i16)
        n245 = Add(x=w386, y=w387) -> (x+y=w385:i16)
        n246 = call <vilib>:"NT Write Number.vi"("Numeric"=w385, "Name"=w384) -> ()  [unwired: 9 in, 1 out]
      }
      event "Test Ring": Value Change {
        n247 = event-data() -> ("NewVal"=w394:u16)  [unwired: 1 in]
        n248 = property on="Test Ring" class="Ring (strict)"() -> ("Strings []"=w395:string[])  [unwired: 2 in, 2 out]
        n249 = Index Array(array=w395, index=w394) -> (element=w393:string)
        n250 = call <vilib>:"NT Write String.vi"("String"=w393, "Name"=w392) -> ()  [unwired: 9 in, 1 out]
      }
      event "Rec Mode": Value Change {
        # "Update globals for recording mode and path to read log from.\nClear when logging and let NetworkTables set path for vision to\nuse."
        n251 = event-data() -> ("NewVal"=w405:enum32{"Stop", "Record", "Playback"})  [unwired: 1 in]
        n252 = global write "WPI_DashboardLogging Global.vi" "Logging Filename"(path "") -> ()
        n253 = case shown="\"Stop\", \"Record\"" w405 {
          tunnel: w404 -> [_ w407 w415]
          tunnel: [_ _ w414] -> w401
          tunnel: [_ _ w413] -> _
          tunnel: w399 -> [_ _ w411]
          tunnel: cluster{i32, i32} {-250, 170} -> [_ _ w410]
          tunnel: [_ _ T21 {"Image Size"=TRUE, "Image Type"=TRUE, "Pixel Value"=TRUE, "ROI Information"=TRUE, "Zoom Factor"=FALSE} ("Image Information Shown:All Elements")] -> w397
          tunnel: [_ _ TRUE ("Zoom Factor")] -> w396
          frame Default {
          }
          frame "Stop", "Record" {
            # "Place Window too"
            n254 = invoke class="VI" method="FP.Close"(reference=w407) -> (reference out=w406:refnum<vi>)  [unwired: 2 in, 2 out]
            n255 = invoke class="VI" method="Abort VI"(reference=w406) -> ()  [unwired: 2 in, 3 out]
          }
          frame "Playback" {
            n256 = call "Open Playback Panel.vi"("Offset"=w410, "DB VI Ref"=w411, "Playback in"=w415) -> ("Playback out"=w412:refnum<vi>)  [unwired: 8 in]
            n257 = register-events(w412) -> (reference out=w414:refnum<event-registration>, error out=w413:errorcluster)  [unwired: 2 in]
          }
        }
        n258 = global write "WPI_DashboardLogging Global.vi" "Recording"(w405) -> ()
        n259 = property on="Camera Image" class="ImageControl"("Image Information Shown"=w397, "Image Information Visible"=w396) -> ()  [unwired: 2 in, 2 out]
        n260 = call <vilib>:"WPI_DashboardNT Log FieldName Cache.vi"("Operation"=enum16{"Lookup/Add", "Index", "Clear"}."Clear") -> ()  [unwired: 8 in, 3 out]
      }
      event Panel Close {
        w416 = enum32{"Stop", "Record", "Playback"}."Stop" ("Rec Mode")
        n261 = event-data() -> ()  [unwired: 1 in, 4 out]
        n262 = local write "Rec Mode"(w416) -> ()
        n263 = global write "WPI_DashboardLogging Global.vi" "Recording"(w416) -> ()
      }
      event Panel Close {
        # "Abort playback window and ourself"
        n264 = event-data() -> ()  [unwired: 1 in, 4 out]
        n265 = invoke class="VI" method="FP.Close"(reference=w421) -> (reference out=w420:refnum<vi>)  [unwired: 2 in, 2 out]
        n266 = invoke class="VI" method="Abort VI"(reference=w420) -> (error out=w419:errorcluster)  [unwired: 2 in, 2 out]
        n267 = invoke class="VI" method="Abort VI"(error in=w419) -> ()  [unwired: 2 in, 3 out]
      }
    }
  }
  n268 = property on="On/Off" class="Bool (strict)"("Visible"=w25) -> ()  [unwired: 2 in, 2 out]
  n269 = property on="Motor" class="Clust (strict)"("Visible"=w25) -> ()  [unwired: 2 in, 2 out]
  n270 = property on="Progress" class="Clust (strict)"("Visible"=w25) -> ()  [unwired: 2 in, 2 out]
  n271 = property on="Test Ring" class="Ring (strict)"("Visible"=w25) -> ()  [unwired: 2 in, 2 out]
  n272 = property on="Rev/Fwd" class="Clust (strict)"("Visible"=w25) -> ()  [unwired: 2 in, 2 out]
  n273 = property on="Camera Settings" class="Clust (strict)"("Visible"=w25) -> ()  [unwired: 2 in, 2 out]
  n274 = local write "DB Camera Config"(w25) -> ()
  n275 = global write "WPI_DashboardLogging Global.vi" "Recording"(w8) -> ()
  n276 = local write "Rec Mode"(w8) -> ()
